vi "Periodic Tasks.vi"(8 "error in":errorcluster) -> ()   [LabVIEW 2013]
doc: "This VI runs in parallel to other tasks. It can contain as many user-defined periodic loops as you need. These can carry out PID or other sorts of timed response."
uses:
  <vilib>/Rock Robotics/SystemInterfaces/Utilities/FPGA_UtilitiesLED Source.ctl
  <vilib>/Rock Robotics/SystemInterfaces/Utilities/FPGA_UtilitiesLED State.ctl
  Robot Global Data.vi
  <vilib>/Rock Robotics/WPI/Compressor/WPI_CompressorGetSetRefNum.vi
panel:
  out "Shoulder Position (%)":dbl
  in  "Shoulder Top (v)":dbl=3.12
  in  "Shoulder Bottom (v)":dbl=1.0
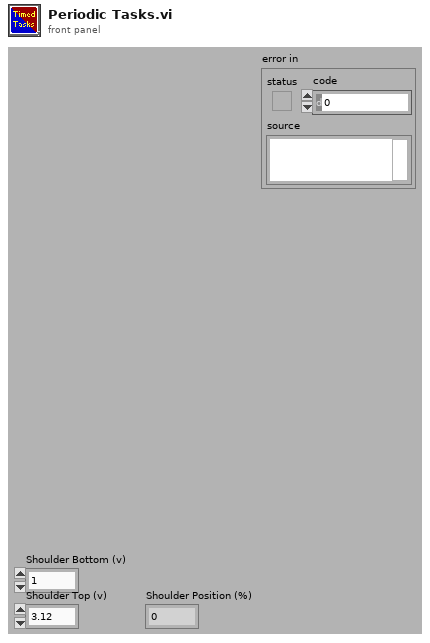
[diagram p1: front panel]
types:
  T1 = typedef "WPI_AnalogChannelDevRef.ctl" = cluster{"DevStatus":errorcluster, "Analog Module":T2, "Analog Channel":T3}
  T2 = typedef "FPGA_TypedefAnalogModule.ctl" = enum16{"Analog Module 1", "Analog Module 2"}
  T3 = typedef "FPGA_AIChannel.ctl" = enum8{"AI 1", "AI 2", "AI 3", "AI 4", "AI 5", "AI 6", "AI 7", "AI 8", "Invalid"}
  T4 = typedef "FPGA_UtilitiesLED State.ctl" = enum16{"Off", "On", "Toggle"}
  T5 = typedef "FPGA_UtilitiesLED Source.ctl" = enum16{"User LED", "FPGA LED"}
  T6 = typedef "WPI_CompressorDevRef.ctl" = cluster{"DevStatus":errorcluster, "DigitalInputDevRef":T7, "RelayDevRef":T10}
  T7 = typedef "WPI_DigitalInputDevRef.ctl" = cluster{"DevStatus":errorcluster, "DIO Channel":T8, "Digital Module":T9}
  T8 = typedef "FPGA_DIOChannel.ctl" = enum8{"DIO 1", "DIO 2", "DIO 3", "DIO 4", "DIO 5", "DIO 6", "DIO 7", "DIO 8", "DIO 9", "DIO 10", "DIO 11", "DIO 12", "DIO 13", "DIO 14", "Invalid"}
  T9 = typedef "FPGA_TypedefDigitalModule.ctl" = enum16{"Digital Module 1", "Digital Module 2"}
  T10 = typedef "WPI_RelayDevRef.ctl" = cluster{"DevStatus":errorcluster, "Relay Channel":T11, "Digital Module":T9, "Relay Direction":T12}
  T11 = typedef "FPGA_DIORelayChannel.ctl" = enum8{"Relay 1", "Relay 2", "Relay 3", "Relay 4", "Relay 5", "Relay 6", "Relay 7", "Relay 8", "Invalid"}
  T12 = typedef "WPI_RelayDirection.ctl" = enum16{"Both directions", "Forward only", "Reverse only"}
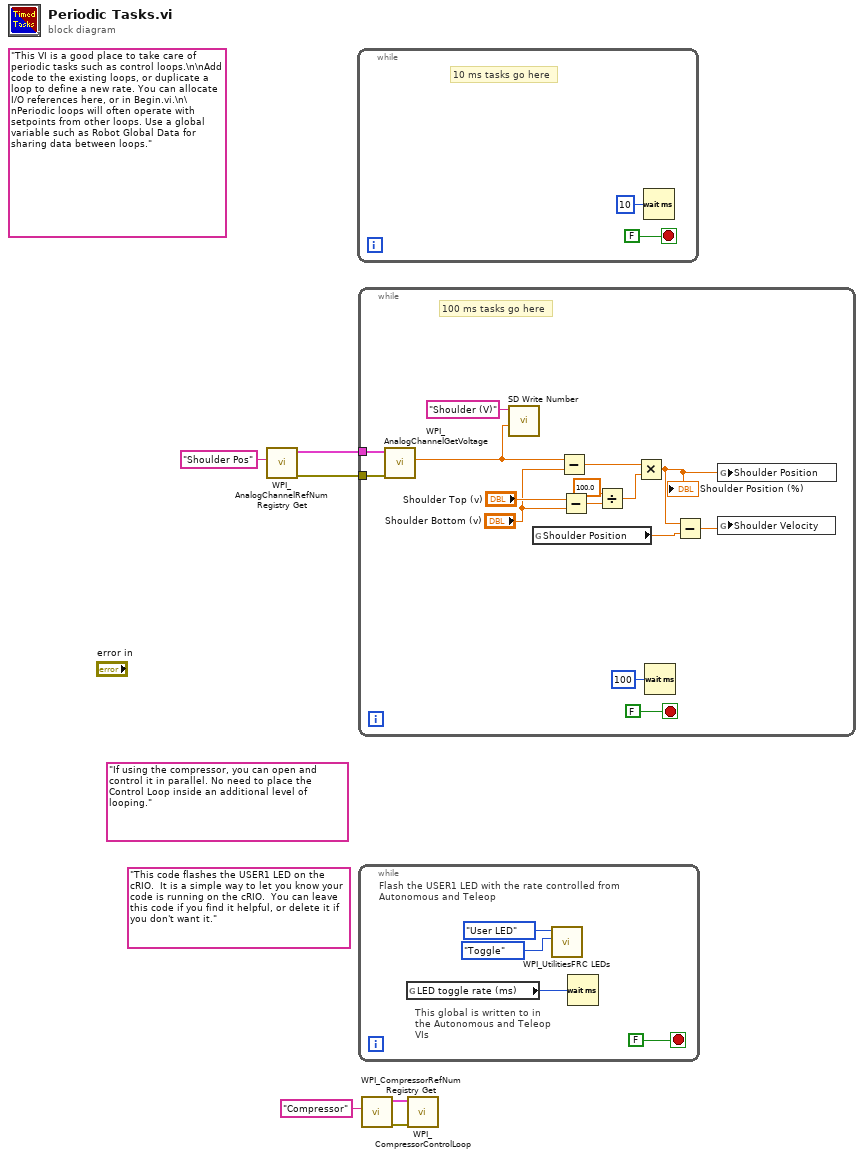
[diagram p0: block diagram]
diagram:
  (unwired) "If using the compressor, you can open and control it in parallel. No need to place the Control Loop inside an additional level of looping."
  (unwired) "This code flashes the USER1 LED on the cRIO.  It is a simple way to let you know your code is running on the cRIO.  You can leave this code if you find it helpful, or delete it if you don't want it."
  (unwired) "This VI is a good place to take care of periodic tasks such as control loops.\n\nAdd code to the existing loops, or duplicate a loop to define a new rate. You can allocate I/O references here, or in Begin.vi.\n\nPeriodic loops will often operate with setpoints from other loops. Use a global variable such as Robot Global Data for sharing data between loops."
  n1 = call <vilib>:"WPI_AnalogChannelRefNum Registry Get.vi"("refnum name"="Shoulder Pos") -> ("error out"=w1:errorcluster, "AIDeviceRef"=w2:T1)  [unwired: 9 in]
  n2 = while {
    stop <- FALSE stop-if-true
    # "10 ms tasks go here"
    n3 = Wait (ms)(milliseconds to wait=u32 10) -> ()  [unwired: 1 out]
  }
  n4 = while {
    tunnel: w2 -> [w21]
    tunnel: w1 -> [w20]
    stop <- FALSE stop-if-true
    # "100 ms tasks go here"
    n5 = call <vilib>:"WPI_AnalogChannelGetVoltage.vi"("error in (no error)"=w20, "AIDeviceRef"=w21) -> ("Voltage"=w10:dbl)  [unwired: 7 in, 2 out]
    n6 = call <vilib>:"SD Write Number.vi"("Numeric"=w10, "Name"="Shoulder (V)") -> ()  [unwired: 8 in, 2 out]
    n7 = global read "Robot Global Data.vi" "Shoulder Position"() -> (w12:dbl)
    n8 = Subtract(x=w10, y="Shoulder Bottom (v)") -> (x-y=w19:dbl)
    n9 = Subtract(x="Shoulder Top (v)", y="Shoulder Bottom (v)") -> (x-y=w17:dbl)
    n10 = Divide(x=100.0, y=w17) -> (x/y=w16:dbl)
    n11 = Multiply(x=w19, y=w16) -> (x*y=w13:dbl)
    "Shoulder Position (%)" <- w13
    n12 = Wait (ms)(milliseconds to wait=u32 100) -> ()  [unwired: 1 out]
    n13 = Subtract(x=w13, y=w12) -> (x-y=w11:dbl)
    n14 = global write "Robot Global Data.vi" "Shoulder Position"(w13) -> ()
    n15 = global write "Robot Global Data.vi" "Shoulder Velocity"(w11) -> ()
  }
  n16 = while {
    stop <- FALSE stop-if-true
    # "This global is written to in the Autonomous and Teleop VIs"
    # "Flash the USER1 LED with the rate controlled from Autonomous and Teleop"
    n17 = global read "Robot Global Data.vi" "LED toggle rate (ms)"() -> (w24:u32)
    n18 = call <vilib>:"WPI_UtilitiesFRC LEDs.vi"("State"=FPGA_UtilitiesLED_State."Toggle", "LED Type"=FPGA_UtilitiesLED_Source."User LED") -> ()  [unwired: 1 in, 9 out]
    n19 = Wait (ms)(milliseconds to wait=w24) -> ()  [unwired: 1 out]
  }
  n20 = call <vilib>:"WPI_CompressorRefNum Registry Get.vi"("refnum name"="Compressor") -> ("error out"=w6:errorcluster, "CompressorDevRef"=w5:T6)  [unwired: 9 in]
  n21 = call <vilib>:"WPI_CompressorControlLoop.vi"("error in (no error)"=w6, "CompressorDevRef"=w5) -> ()  [unwired: 10 in]
